vi "mod_control changed(array).vi"(2 "refnum array":refnum<vi>[](array[refnum]), 4 "initialize?":bool) -> (7 "changed?":bool)   [LabVIEW 2020, in "niAMT.lvlib"]
uses:
  <vilib>/addons/Modulation/niAMT.lvlib
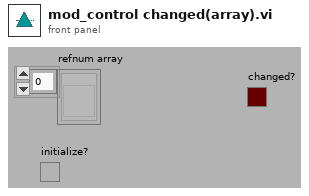
[diagram p1: front panel]
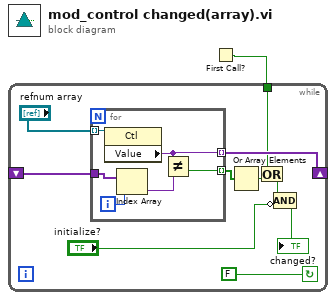
[diagram p0: block diagram]
diagram:
  n1 = First Call?() -> (First Call?: T/F=w1:bool)
  n2 = while {
    tunnel: w1 -> [w2]
    shift-left: _ -> [w8]
    shift-right: [w9] -> _
    stop <- FALSE continue-if-true
    n3 = for {
      tunnel: "refnum array" -> [w17] mode=indexing
      tunnel: [w16] -> w9 mode=indexing
      tunnel: w8 -> [w15]
      tunnel: [w14] -> w7 mode=indexing
      i -> [w12]
      n4 = property class="Ctl"(reference=w17) -> ("Value"=w16:variant)  [unwired: 1 in, 2 out]
      n5 = Index Array(array=w15, index=w12) -> (element=w13:variant)
      n6 = Not Equal?(x=w16, y=w13) -> (x != y?=w14:bool)
    }
    n7 = Or Array Elements(Boolean array=w7) -> (logical OR=w3:bool)
    n8 = Or(x=w2, y=w3) -> (x .or. y?=w4:bool)
    n9 = Compound Arithmetic op=AND(w4, invert "initialize?") -> (→"changed?":bool)
  }
